vi "Block Size From Speed.vi"(4 "speed (rpm)":dbl) -> (1 "block size (sec)":dbl)   [LabVIEW 2017, in "VibrationAnalysisFunctions.lvlib"]
uses:
  <vilib>/addons/InsightCM/Utilities/Analysis/Vibration/VibrationAnalysisFunctions.lvlib
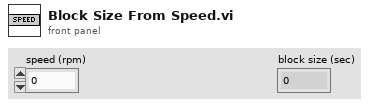
[diagram p1: front panel]
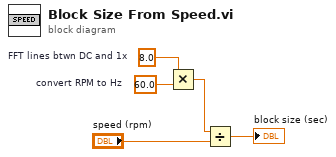
[diagram p0: block diagram]
diagram:
  w4 = 8.0  # FFT lines btwn DC and 1x
  w5 = 60.0  # convert RPM to Hz
  n1 = Multiply(x=w4, y=w5) -> (x*y=w3:dbl)
  n2 = Divide(x=w3, y="speed (rpm)") -> (x/y=→"block size (sec)":dbl)
